vi "onHttpPost (File).vi"(6 "timeout":i32=10000, 7 "output file":path, 8 "error in":errorcluster, 9 "file":path, 10 "url":string, 11 "http-method in":refnum<class "REST Client.lvclass">) -> (0 "error out":errorcluster, 1 "body":string, 2 "headers":string, 3 "http-method out":refnum<class "REST Client.lvclass">)   [LabVIEW 2020, in "REST Client.lvlib" / "REST Client.lvclass"]
uses:
  REST Client.lvclass
  REST Client.lvclass/REST Client.ctl
  http-client/http-client.lvclass
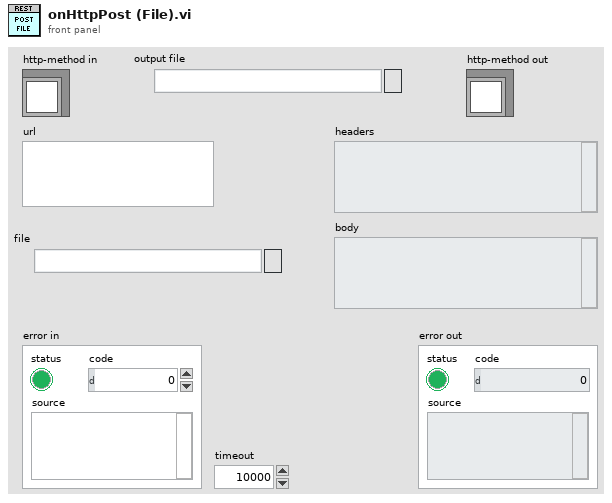
[diagram p1: front panel]
types:
  T1 = typedef "REST Client.lvlib/REST Client.lvclass/HTTP Header.ctl" = cluster{"header":T2, "value":string}
  T2 = typedef "lib_NI_Advanced HTTP Client.lvlib/Session.lvclass/Header--Combo Box.ctl" = string
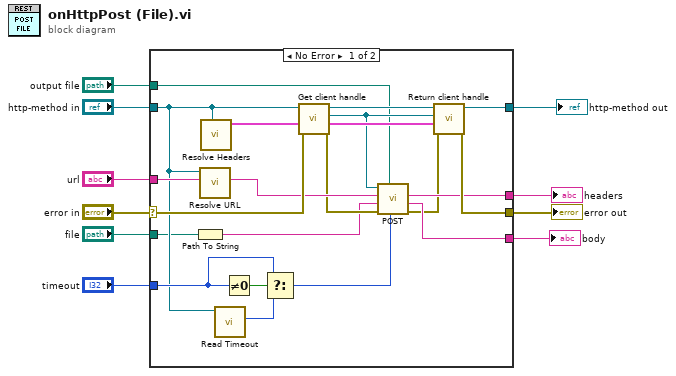
[diagram p0: block diagram]
diagram:
  n1 = case shown="No Error" "error in" {
    selector: "error in" -> [w25 w33]
    tunnel: [w21 w33] -> w6
    tunnel: [w22 w32] -> w9
    tunnel: "http-method in" -> [w24 w32]
    tunnel: "url" -> [w29 _]
    tunnel: "timeout" -> [w27 _]
    tunnel: [w18 _] -> w7
    tunnel: [w17 _] -> w8
    tunnel: "output file" -> [w15 _]
    tunnel: "file" -> [w12 _]
    frame No Error {
      n2 = Path To String(path=w12) -> (string=w11:string)
      n3 = call "Resolve URL.vi"("Path"=w29, "REST Client in"=w24) -> ("Resolved URL"=w19:string)  [unwired: 9 in]
      n4 = call "Resolve Headers.vi"("REST Client in"=w24) -> ("headers out"=w23:T1[])  [unwired: 10 in]
      n5 = call-dynamic "Read Timeout.vi"("REST Client in"=w24) -> ("Timeout"=w26:i32)  [unwired: 8 in, 2 out]
      n6 = Not Equal To 0?(x=w27) -> (x != 0?=w28:bool)
      n7 = Select(t=w27, s=w28, f=w26) -> (s? t:f=w13:i32)
      n8 = call "Get client handle.vi"("error in (no error)"=w25, "headers"=w23, "REST Client in"=w24) -> ("error out"=w14:errorcluster, "headers out"=w30:T1[], "http-client"=w20:refnum<class "http-client.lvclass">, "REST Client out"=w31:refnum<class "REST Client.lvclass">)  [unwired: 5 in]
      n9 = call "POST.vi"("timeout"=w13, "output file"=w15, "error in"=w14, "buffer"=w11, "url"=w19, "http-client in"=w20) -> ("error out"=w16:errorcluster, "body"=w17:string, "headers"=w18:string)  [unwired: 1 in, 2 out]
      n10 = call "Return client handle.vi"("error in (no error)"=w16, "headers"=w30, "http-client"=w20, "REST Client in"=w31) -> ("error out"=w21:errorcluster, "REST Client out"=w22:refnum<class "REST Client.lvclass">)  [unwired: 6 in]
    }
    frame Error {
    }
  }
  "error out" <- w6
  "http-method out" <- w9
  "headers" <- w7
  "body" <- w8
